vi "daqio_Create_Default_Dashboard.vi"(8 "error in (no error)":errorcluster, 11 "daq.io type in":T2={"daq.io ref"=refnum, "daq.io API Base"="http://dashboard.daq.io/api/v1", "Device Type Key"="", "Device Key"="", "Account ID"=""}) -> (0 "error out":errorcluster, 1 "Dashboard URL":string, 2 "Dashboard return":T1, 3 "daq.io type out":T2={"daq.io ref"=refnum, "daq.io API Base"="http://dashboard.daq.io/api/v1", "Device Type Key"="", "Device Key"="", "Account ID"=""})   [LabVIEW 2013, in "daqio minimal.lvlib"]
doc: "This VI creates a new default dashboard for a specific account and makes it the new default dashboard for the current device."
uses:
  daqio minimal.lvlib
  _typedefs/daqio-Type.ctl
  <vilib>/httpClient/ClientHandle.ctl
  _typedefs/daqio-Device_w_Dashboard.ctl
  <vilib>/Easy HTTP Client/Easy HTTP.lvlib
  <vilib>/httpClient/LabVIEWHTTPClient.lvlib
panel:
  out "body":string
  out "JSON string":string
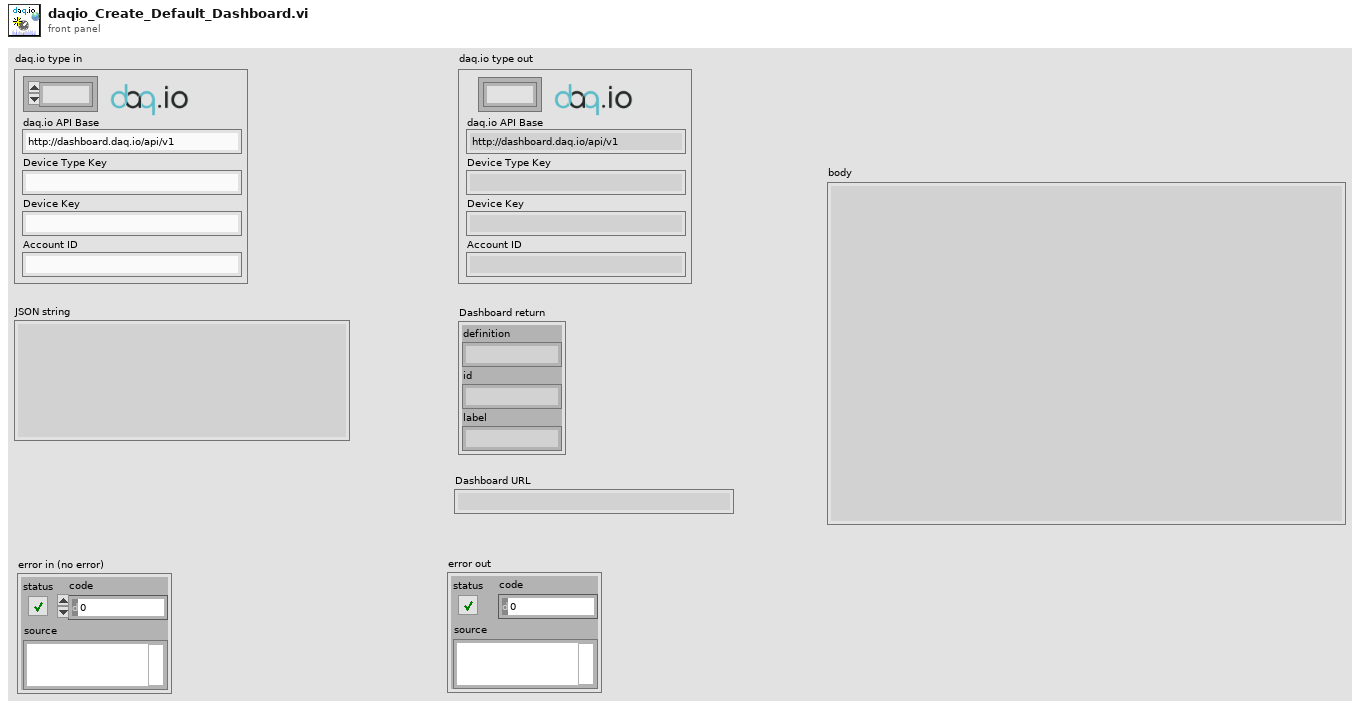
[diagram p1: front panel]
types:
  T1 = cluster{"definition":string, "id":string, "label":string}
  T2 = typedef "daqio minimal.lvlib/daqio-Type.ctl" = cluster{"daq.io ref":T3, "daq.io API Base":string, "Device Type Key":string, "Device Key":string, "Account ID":string}
  T3 = typedef "LabVIEWHTTPClient.lvlib/ClientHandle.ctl" = refnum<k1>
  T4 = typedef "daqio minimal.lvlib/daqio-Device_w_Dashboard.ctl" = cluster{"permissions":cluster{"write":string[], "read":string[]}, "id":string, "label":string, "key":string, "device_type_id":string, "tags":cluster{"key":string, "value":string}[], "assets":string[], "default_dashboard_id":string}
  T5 = typedef "daqio minimal.lvlib/daqio-Channel-Type-POST-return.ctl" = cluster{"device_type_id":string, "id":string, "key":string, "label":string, "data_type":string, "permissions":cluster{"write":string[], "read":string[]}}
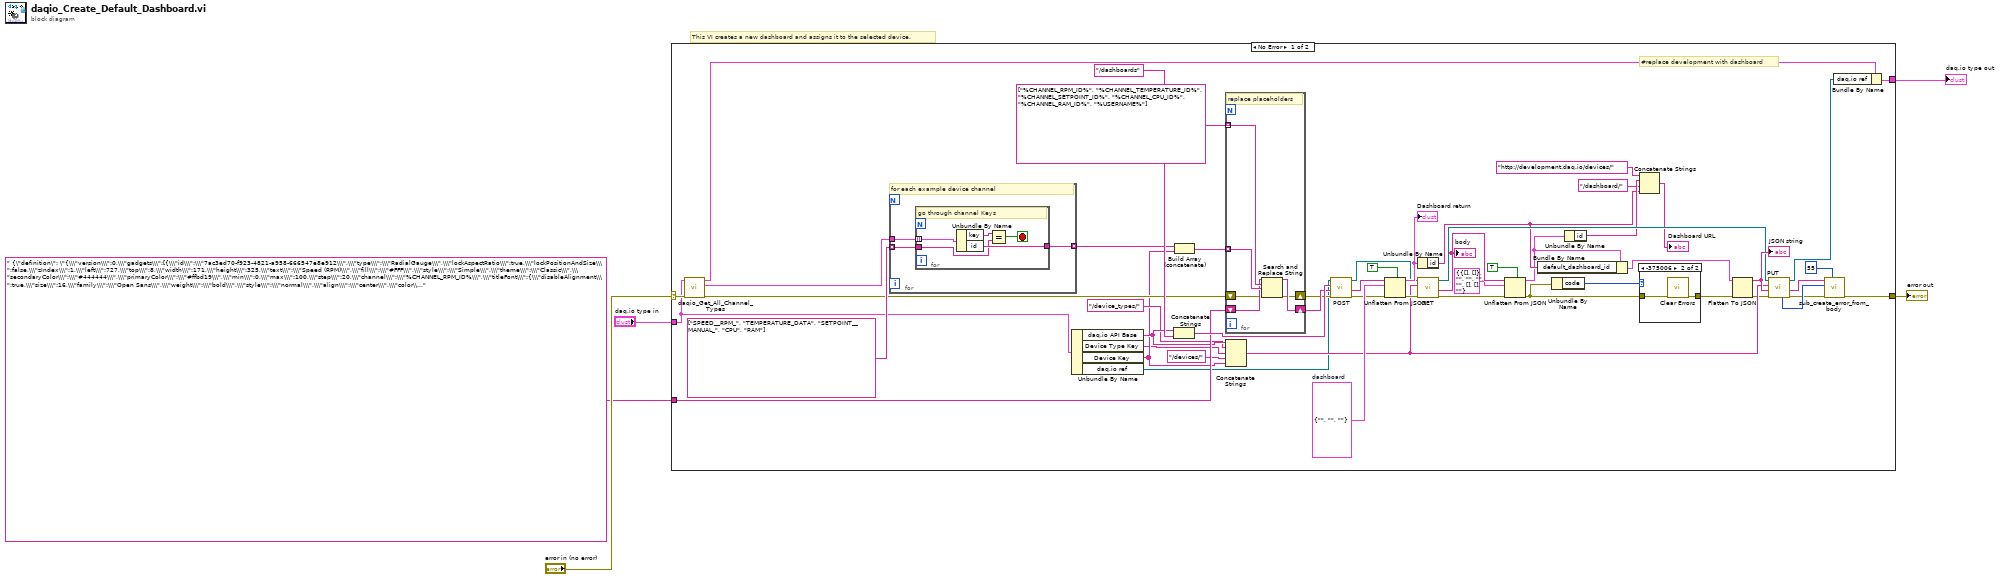
[diagram p0: block diagram]
diagram:
  # "This VI creates a new dashboard and assigns it to the selected device."
  n1 = case shown="No Error" "error in (no error)" {
    selector: "error in (no error)" -> [w55 w75]
    tunnel: "daq.io type in" -> [w46 w76]
    tunnel: [w54 w76] -> w4
    tunnel: [w22 w75] -> w3
    tunnel: " {\"definition\": \"{\\\"version\\\":0,\\\"gadgets\\\":[{\\\"id\\\":\\\"7ac3ed70-f923-4821-a958-666547e8e912\\\",\\\"type\\\":\\\"RadialGauge\\\",\\\"lockAspectRatio\\\":true,\\\"lockPositionAndSize\\\":false,\\\"zIndex\\\":1,\\\"left\\\":727,\\\"top\\\":8,\\\"width\\\":171,\\\"height\\\":325,\\\"text\\\":\\\"Speed (RPM)\\\",\\\"fill\\\":\\\"#FFF\\\",\\\"style\\\":\\\"Simple\\\",\\\"theme\\\":\\\"Classic\\\",\\\"secondaryColor\\\":\\\"#444444\\\",\\\"primaryColor\\\":\\\"#ffbd19\\\",\\\"min\\\":0,\\\"max\\\":100,\\\"step\\\":20,\\\"channel\\\":\\\"%CHANNEL_RPM_ID%\\\",\\\"titleFont\\\":{\\\"disableAlignment\\\":true,\\\"size\\\":16,\\\"family\\\":\\\"Open Sans\\\",\\\"weight\\\":\\\"bold\\\",\\\"style\\\":\\\"normal\\\",\\\"align\\\":\\\"center\\\",\\\"color\\\":\\\"#777\\\",\\\"drawBoxesAroundText\\\":false,\\\"sizeLocked\\\":true},\\\"unitFont\\\":{\\\"disableAlignment\\\":true,\\\"size\\\":0,\\\"family\\\":\\\"Open Sans\\\",\\\"weight\\\":\\\"normal\\\",\\\"style\\\":\\\"normal\\\",\\\"align\\\":\\\"center\\\",\\\"color\\\":\\\"#777\\\",\\\"drawBoxesAroundText\\\":false},\\\"valueFont\\\":{\\\"disableAlignment\\\":true,\\\"size\\\":26.71875,\\\"family\\\":\\\"Open Sans\\\",\\\"weight\\\":\\\"bold\\\",\\\"style\\\":\\\"normal\\\",\\\"align\\\":\\\"center\\\",\\\"color\\\":\\\"#777\\\",\\\"drawBoxesAroundText\\\":false},\\\"rangeFont\\\":{\\\"disableAlignment\\\":true,\\\"size\\\":10.6875,\\\"family\\\":\\\"Open Sans\\\",\\\"weight\\\":\\\"normal\\\",\\\"style\\\":\\\"normal\\\",\\\"align\\\":\\\"center\\\",\\\"color\\\":\\\"#777\\\"}},{\\\"id\\\":\\\"7e0172ce-b84d-437a-9326-f0fd3ac7a2ed\\\",\\\"type\\\":\\\"Image\\\",\\\"lockAspectRatio\\\":true,\\\"lockPositionAndSize\\\":false,\\\"zIndex\\\":1,\\\"left\\\":376,\\\"top\\\":211,\\\"width\\\":222,\\\"height\\\":147,\\\"image\\\":\\\"https://daqio-assets.s3.amazonaws.com/centrifuge_original.png\\\"},{\\\"id\\\":\\\"4d953908-15d4-4226-91de-77cd2beb7e82\\\",\\\"type\\\":\\\"Shape\\\",\\\"lockAspectRatio\\\":true,\\\"lockPositionAndSize\\\":false,\\\"zIndex\\\":0,\\\"left\\\":362,\\\"top\\\":138,\\\"width\\\":254,\\\"height\\\":254,\\\"shape\\\":\\\"Circle\\\",\\\"strokeWidth\\\":\\\"1\\\",\\\"stroke\\\":\\\"#7a7a7a\\\",\\\"fill\\\":\\\"#e1e1e1\\\"},{\\\"id\\\":\\\"c9c26b4d-9cbf-4a0a-b91e-2f65f7344d33\\\",\\\"type\\\":\\\"Label\\\",\\\"lockAspectRatio\\\":true,\\\"lockPositionAndSize\\\":false,\\\"zIndex\\\":0,\\\"left\\\":350,\\\"top\\\":-47,\\\"width\\\":300,\\\"height\\\":250,\\\"text\\\":\\\"Centrifuge Demo\\\",\\\"contentFont\\\":{\\\"size\\\":20,\\\"family\\\":\\\"Open Sans\\\",\\\"weight\\\":\\\"bold\\\",\\\"style\\\":\\\"normal\\\",\\\"align\\\":\\\"center\\\",\\\"color\\\":\\\"#000000\\\",\\\"drawBoxesAroundText\\\":true,\\\"colorLocked\\\":true}},{\\\"id\\\":\\\"7e77ffad-4046-414f-a2d7-29a2a5b95539\\\",\\\"type\\\":\\\"HorizontalChart\\\",\\\"lockAspectRatio\\\":false,\\\"lockPositionAndSize\\\":false,\\\"zIndex\\\":0,\\\"left\\\":44,\\\"top\\\":472,\\\"width\\\":886,\\\"height\\\":251,\\\"channels\\\":[\\\"%CHANNEL_TEMPERATURE_ID%\\\"],\\\"chartType\\\":\\\"Line\\\",\\\"title\\\":\\\"Live Data\\\",\\\"animation\\\":false,\\\"bezierCurve\\\":false,\\\"showScale\\\":true,\\\"showScaleLabels\\\":true,\\\"fillColor\\\":\\\"rgba(151,187,205,0.2)\\\",\\\"strokeColor\\\":\\\"rgba(151,187,205,1)\\\",\\\"pointColor\\\":\\\"rgba(151,187,205,1)\\\",\\\"pointDot\\\":false,\\\"datasetFill\\\":false},{\\\"id\\\":\\\"6d40786f-8469-407d-82b0-a8fb2274aa41\\\",\\\"type\\\":\\\"Label\\\",\\\"lockAspectRatio\\\":false,\\\"lockPositionAndSize\\\":false,\\\"zIndex\\\":0,\\\"left\\\":383,\\\"top\\\":406,\\\"width\\\":200,\\\"height\\\":67,\\\"text\\\":\\\"Temperature\\\",\\\"contentFont\\\":{\\\"size\\\":13,\\\"family\\\":\\\"Open Sans\\\",\\\"weight\\\":\\\"normal\\\",\\\"style\\\":\\\"normal\\\",\\\"align\\\":\\\"center\\\",\\\"color\\\":\\\"#777\\\",\\\"drawBoxesAroundText\\\":false,\\\"sizeLocked\\\":true}},{\\\"id\\\":\\\"cb40a290-c180-4a08-89c5-431a35526d9e\\\",\\\"type\\\":\\\"HorizontalBar\\\",\\\"lockAspectRatio\\\":true,\\\"lockPositionAndSize\\\":false,\\\"zIndex\\\":0,\\\"left\\\":10,\\\"top\\\":111,\\\"width\\\":300,\\\"height\\\":100,\\\"text\\\":\\\"CPU\\\",\\\"style\\\":\\\"Simple\\\",\\\"theme\\\":\\\"Outline\\\",\\\"min\\\":0,\\\"max\\\":100,\\\"titleFont\\\":{\\\"size\\\":18,\\\"family\\\":\\\"Open Sans\\\",\\\"weight\\\":\\\"bold\\\",\\\"style\\\":\\\"normal\\\",\\\"align\\\":\\\"center\\\",\\\"color\\\":\\\"#777\\\",\\\"drawBoxesAroundText\\\":false},\\\"unitFont\\\":{\\\"size\\\":0,\\\"family\\\":\\\"Open Sans\\\",\\\"weight\\\":\\\"normal\\\",\\\"style\\\":\\\"normal\\\",\\\"align\\\":\\\"center\\\",\\\"color\\\":\\\"#777\\\",\\\"drawBoxesAroundText\\\":false},\\\"valueFont\\\":{\\\"size\\\":20,\\\"family\\\":\\\"Open Sans\\\",\\\"weight\\\":\\\"bold\\\",\\\"style\\\":\\\"normal\\\",\\\"align\\\":\\\"center\\\",\\\"color\\\":\\\"#999999\\\",\\\"drawBoxesAroundText\\\":false,\\\"colorLocked\\\":true},\\\"rangeFont\\\":{\\\"size\\\":16,\\\"family\\\":\\\"Open Sans\\\",\\\"weight\\\":\\\"normal\\\",\\\"style\\\":\\\"normal\\\",\\\"align\\\":\\\"center\\\",\\\"color\\\":\\\"#777\\\",\\\"drawBoxesAroundText\\\":false},\\\"barColor\\\":\\\"#ffd231\\\",\\\"channel\\\":\\\"%CHANNEL_CPU_ID%\\\"},{\\\"id\\\":\\\"6f7b8051-d386-4202-81a3-3c12b381a257\\\",\\\"type\\\":\\\"HorizontalBar\\\",\\\"lockAspectRatio\\\":true,\\\"lockPositionAndSize\\\":false,\\\"zIndex\\\":0,\\\"left\\\":6,\\\"top\\\":220,\\\"width\\\":300,\\\"height\\\":100,\\\"text\\\":\\\"RAM\\\",\\\"style\\\":\\\"Simple\\\",\\\"theme\\\":\\\"Outline\\\",\\\"min\\\":0,\\\"max\\\":100,\\\"titleFont\\\":{\\\"size\\\":18,\\\"family\\\":\\\"Open Sans\\\",\\\"weight\\\":\\\"bold\\\",\\\"style\\\":\\\"normal\\\",\\\"align\\\":\\\"center\\\",\\\"color\\\":\\\"#777\\\",\\\"drawBoxesAroundText\\\":false},\\\"unitFont\\\":{\\\"size\\\":0,\\\"family\\\":\\\"Open Sans\\\",\\\"weight\\\":\\\"normal\\\",\\\"style\\\":\\\"normal\\\",\\\"align\\\":\\\"center\\\",\\\"color\\\":\\\"#777\\\"},\\\"valueFont\\\":{\\\"size\\\":20,\\\"family\\\":\\\"Open Sans\\\",\\\"weight\\\":\\\"bold\\\",\\\"style\\\":\\\"normal\\\",\\\"align\\\":\\\"center\\\",\\\"color\\\":\\\"#979797\\\",\\\"drawBoxesAroundText\\\":false,\\\"colorLocked\\\":true},\\\"rangeFont\\\":{\\\"size\\\":16,\\\"family\\\":\\\"Open Sans\\\",\\\"weight\\\":\\\"normal\\\",\\\"style\\\":\\\"normal\\\",\\\"align\\\":\\\"center\\\",\\\"color\\\":\\\"#777\\\",\\\"drawBoxesAroundText\\\":false},\\\"barColor\\\":\\\"#ffd231\\\",\\\"channel\\\":\\\"%CHANNEL_RAM_ID%\\\"},{\\\"id\\\":\\\"6e31d9f8-654d-4a90-a645-4c0c01ffefb2\\\",\\\"type\\\":\\\"RadialGauge\\\",\\\"lockAspectRatio\\\":true,\\\"lockPositionAndSize\\\":false,\\\"zIndex\\\":1,\\\"left\\\":729,\\\"top\\\":197,\\\"width\\\":171,\\\"height\\\":325,\\\"text\\\":\\\"Setpoint\\\",\\\"fill\\\":\\\"#FFF\\\",\\\"style\\\":\\\"Simple\\\",\\\"theme\\\":\\\"Classic\\\",\\\"secondaryColor\\\":\\\"#444444\\\",\\\"primaryColor\\\":\\\"#ffbd19\\\",\\\"min\\\":0,\\\"max\\\":100,\\\"step\\\":20,\\\"channel\\\":\\\"%CHANNEL_SETPOINT_ID%\\\",\\\"titleFont\\\":{\\\"disableAlignment\\\":true,\\\"size\\\":16,\\\"family\\\":\\\"Open Sans\\\",\\\"weight\\\":\\\"bold\\\",\\\"style\\\":\\\"normal\\\",\\\"align\\\":\\\"center\\\",\\\"color\\\":\\\"#777\\\",\\\"drawBoxesAroundText\\\":false,\\\"sizeLocked\\\":true},\\\"unitFont\\\":{\\\"disableAlignment\\\":true,\\\"size\\\":0,\\\"family\\\":\\\"Open Sans\\\",\\\"weight\\\":\\\"normal\\\",\\\"style\\\":\\\"normal\\\",\\\"align\\\":\\\"center\\\",\\\"color\\\":\\\"#777\\\",\\\"drawBoxesAroundText\\\":false},\\\"valueFont\\\":{\\\"disableAlignment\\\":true,\\\"size\\\":26.71875,\\\"family\\\":\\\"Open Sans\\\",\\\"weight\\\":\\\"bold\\\",\\\"style\\\":\\\"normal\\\",\\\"align\\\":\\\"center\\\",\\\"color\\\":\\\"#777\\\",\\\"drawBoxesAroundText\\\":false},\\\"rangeFont\\\":{\\\"disableAlignment\\\":true,\\\"size\\\":10.6875,\\\"family\\\":\\\"Open Sans\\\",\\\"weight\\\":\\\"normal\\\",\\\"style\\\":\\\"normal\\\",\\\"align\\\":\\\"center\\\",\\\"color\\\":\\\"#777\\\"}},{\\\"id\\\":\\\"90ba8f3d-be02-42b1-90c0-ea490e721fa7\\\",\\\"type\\\":\\\"Image\\\",\\\"lockAspectRatio\\\":true,\\\"lockPositionAndSize\\\":false,\\\"zIndex\\\":0,\\\"left\\\":445,\\\"top\\\":12,\\\"width\\\":92,\\\"height\\\":61,\\\"image\\\":\\\"https://daqio-assets.s3.amazonaws.com/daq.io_small.png\\\"},{\\\"id\\\":\\\"03293aae-fb6d-482e-9e2c-42fb101fcfef\\\",\\\"type\\\":\\\"HorizontalChart\\\",\\\"lockAspectRatio\\\":false,\\\"lockPositionAndSize\\\":false,\\\"zIndex\\\":0,\\\"left\\\":49,\\\"top\\\":473,\\\"width\\\":853,\\\"height\\\":219,\\\"channels\\\":[\\\"%CHANNEL_TEMPERATURE_ID%\\\"],\\\"chartType\\\":\\\"Line\\\",\\\"title\\\":\\\"Live Data\\\",\\\"animation\\\":false,\\\"bezierCurve\\\":false,\\\"showScale\\\":true,\\\"showScaleLabels\\\":true,\\\"fillColor\\\":\\\"rgba(151,187,205,0.2)\\\",\\\"strokeColor\\\":\\\"rgba(151,187,205,1)\\\",\\\"pointColor\\\":\\\"rgba(151,187,205,1)\\\",\\\"pointDot\\\":false,\\\"datasetFill\\\":false}],\\\"background\\\":\\\"#FFF\\\",\\\"aspectRatio\\\":\\\"1280x720\\\"}\",\n    \"label\": \"LabVIEW Example %USERNAME%\"\n  }" -> [w50 _]
    frame No Error {
      w41 = T1 {"definition"="", "id"="", "label"=""}  # dashboard
      # "#replace development with dashboard"
      n2 = call "daqio_Get_All_Channel_Types.vi"("error in (no error)"=w55, "daq.io type in"=w46) -> ("error out"=w44:errorcluster, "All Channel Types"=w53:T5[], "daq.io type out"=w45:T2)  [unwired: 7 in]
      n3 = for {
        tunnel: w53 -> [w69]
        tunnel: string[] ["SPEED__RPM_", "TEMPERATURE_DATA", "SETPOINT__MANUAL_", "CPU", "RAM"] -> [w68] mode=indexing
        tunnel: [w67] -> w48 mode=indexing
        # "for each example device channel"
        n4 = for {
          tunnel: [w74] -> w67
          tunnel: w69 -> [w73] mode=indexing
          tunnel: w68 -> [w72]
          stop <- w70 stop-if-true
          # "go through channel Keys"
          n5 = Unbundle By Name(w73) -> ("key"=w71:string, "id"=w74:string)
          n6 = Equal?(x=w71, y=w72) -> (x = y?=w70:bool)
        }
      }
      n7 = Unbundle By Name(w46) -> ("daq.io API Base"=w37:string, "Device Type Key"=w18:string, "Device Key"=w19:string, "daq.io ref"=w21:T3)
      n8 = Concatenate Strings(w37, "/dashboards") -> (w56:string)
      n9 = Build Array (concatenate)(w48, w19) -> (w47:string[])
      n10 = for {
        tunnel: w47 -> [w66] mode=indexing
        tunnel: string[] ["%CHANNEL_RPM_ID%", "%CHANNEL_TEMPERATURE_ID%", "%CHANNEL_SETPOINT_ID%", "%CHANNEL_CPU_ID%", "%CHANNEL_RAM_ID%", "%USERNAME%"] -> [w65] mode=indexing
        shift-right: [w63] -> w49
        shift-left: w50 -> [w64]
        shift-right: [w61] -> w43
        shift-left: w44 -> [w62]
        # "replace placeholders"
        n11 = Search and Replace String(input string=w64, search string=w65, replace string=w66, error in=w62) -> (result string=w63:string, error out=w61:errorcluster)  [unwired: 4 in, 2 out]
      }
      n12 = Concatenate Strings(w37, "/device_types/" ("string"), w18, "/devices/" ("string"), w19) -> (w28:string)
      n13 = call <vilib>:"POST.vi"("error in (no error)"=w43, "data"=w49, "url"=w56, "client handle"=w21) -> ("error out"=w39:errorcluster, "body"=w42:string, "client handle out"=w34:T3)  [unwired: 3 in, 2 out]
      n14 = Unflatten From JSON(enable LabVIEW extensions? (T)=TRUE, JSON string=w42, type and defaults=w41, error in (no error)=w39) -> (value=w38:T1, error out=w33:errorcluster)  [unwired: 3 in]
      "Dashboard return" <- w38
      n15 = Unbundle By Name(w38) -> ("id"=w11:string)
      n16 = call <vilib>:"GET.vi"("error in (no error)"=w33, "url"=w28, "client handle"=w34) -> ("error out"=w31:errorcluster, "body"=w32:string, "client handle out"=w27:T3)  [unwired: 4 in, 2 out]
      "body" <- w32
      n17 = Unflatten From JSON(enable LabVIEW extensions? (T)=TRUE, JSON string=w32, type and defaults=T4 {"permissions"={"write"=[], "read"=[]}, "id"="", "label"="", "key"="", "device_type_id"="", "tags"=[], "assets"=[], "default_dashboard_id"=""} ("Device"), error in (no error)=w31) -> (value=w10:T4, error out=w7:errorcluster)  [unwired: 3 in]
      n18 = Bundle By Name(cluster=w10, "default_dashboard_id"=w11) -> (w12:T4)
      n19 = Unbundle By Name(w7) -> ("code"=w8:i32)
      n20 = Unbundle By Name(w10) -> ("id"=w16:string)
      n21 = Concatenate Strings("http://development.daq.io/devices/" ("string"), w16, "/dashboard/" ("string"), w11) -> (→"Dashboard URL":string)
      n22 = case shown="-375006" w8 {
        tunnel: w7 -> [w58 w60]
        tunnel: [w58 w59] -> w6
        frame 0, Default {
        }
        frame -375006 {
          n23 = call <vilib>:"Clear Errors.vi"("error in (no error)"=w60) -> ("error out"=w59:errorcluster)  [unwired: 6 in]
        }
      }
      n24 = Flatten To JSON(anything=w12, error in (no error)=w6) -> (JSON string=w29:string, 11:w13:errorcluster)  [unwired: 1 in]
      "JSON string" <- w29
      n25 = call <vilib>:"PUT.vi"("error in (no error)"=w13, "data"=w29, "url"=w28, "client handle"=w27) -> ("error out"=w25:errorcluster, "body"=w23:string, "client handle out"=w20:T3, "HTTP Response Code"=w26:i32)  [unwired: 3 in, 1 out]
      n26 = call "sub_create_error_from_body.vi"("error code"=55, "error in (no error)"=w25, "http code"=w26, "body"=w23) -> ("error out"=w22:errorcluster)  [unwired: 7 in]
      n27 = Bundle By Name(cluster=w45, "daq.io ref"=w20) -> (w54:T2)
    }
    frame Error {
    }
  }
  "error out" <- w3
  "daq.io type out" <- w4
